vi "Zero Drive Encoders.vi"   [LabVIEW 2012]
uses:
  Globals/Encoders Global.vi
types:
  T1 = typedef "WPI_EncoderDevRef.ctl" = cluster{"DevStatus":errorcluster, "EncoderIndex":T2, "CounterIndex":T3, "DistancePerCount":dbl, "Decoding Type":T4}
  T2 = typedef "FPGA_EncoderIdx.ctl" = enum8{"Enc 0", "Enc 1", "Enc 2", "Enc 3", "Invalid"}
  T3 = typedef "FPGA_CounterCtrSystemIndex.ctl" = enum8{"Ctr 0", "Ctr 1", "Ctr 2", "Ctr 3", "Ctr 4", "Ctr 5", "Ctr 6", "Ctr 7", "Invalid"}
  T4 = typedef "WPI_EncoderType.ctl" = enum16{"1x", "2x", "4x"}
  T5 = cluster{"Front Left":T1, "Front Right":T1, "Rear Left":T1, "Rear Right":T1, "Shooter":T1}
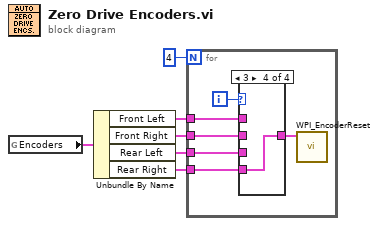
[diagram p0: block diagram]
diagram:
  n1 = global read "Encoders Global.vi" "Encoders"() -> (w5:T5)
  n2 = Unbundle By Name(w5) -> ("Front Left"=w4:T1, "Front Right"=w3:T1, "Rear Left"=w2:T1, "Rear Right"=w1:T1)
  n3 = for {
    N: 4 -> [_]
    tunnel: w4 -> [w11]
    tunnel: w3 -> [w10]
    tunnel: w2 -> [w9]
    tunnel: w1 -> [w8]
    i -> [w12]
    n4 = case shown="3" w12 {
      tunnel: w11 -> [w13 _ _ _]
      tunnel: w10 -> [_ w14 _ _]
      tunnel: w9 -> [_ _ w15 _]
      tunnel: w8 -> [_ _ _ w16]
      tunnel: [w13 w14 w15 w16] -> w7
      frame 0, Default {
      }
      frame 1 {
      }
      frame 2 {
      }
      frame 3 {
      }
    }
    n5 = call <vilib>:"WPI_EncoderReset.vi"("EncoderDevRef"=w7) -> ()  [unwired: 9 in, 2 out]
  }
